vi "Get Row Subset as String Array.vi"(8 "error in (no error)":errorcluster, 9 "Replace FKs?":bool, 10 "Column Names (All)":string[](array[string]), 11 "Basic Table in":refnum<class "Basic Table.lvclass">) -> (0 "error out":errorcluster, 2 "Values":string[](array[string]), 3 "Basic Table out":refnum<class "Basic Table.lvclass">)   [LabVIEW 2020, in "Table.lvlib" / "Basic Table.lvclass"]
uses:
  Basic Table.lvclass
  Basic Table.lvclass/Basic Table.ctl
  Column Libraries/Column Interface/Column Interface Class/Column Interface.lvclass
  Table Configuration Interface/Table Configuration Interface.lvclass
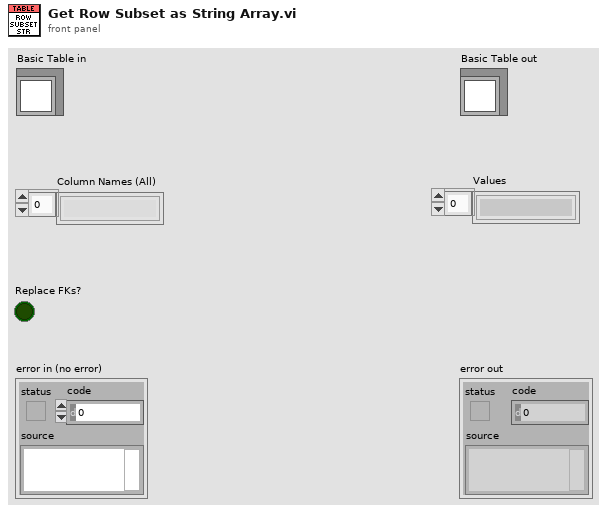
[diagram p1: front panel]
types:
  T1 = map{string, refnum<class "Column Interface.lvclass">}
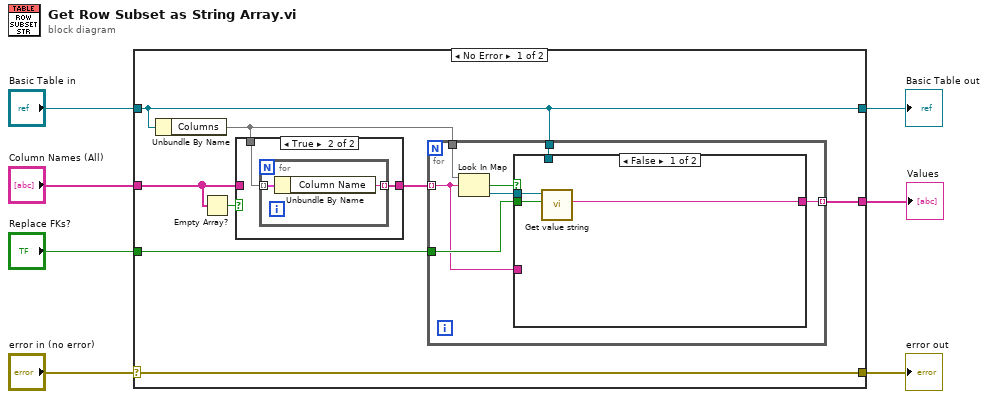
[diagram p0: block diagram]
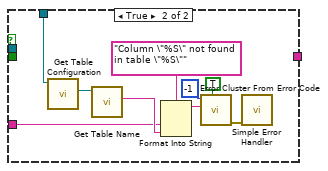
[diagram p3: hidden frame]
diagram:
  n1 = case shown="No Error" "error in (no error)" {
    selector: "error in (no error)" -> [w12 w41]
    tunnel: [w12 w41] -> w6
    tunnel: [w13 w40] -> w4
    tunnel: "Basic Table in" -> [w13 w40]
    tunnel: "Column Names (All)" -> [w10 _]
    tunnel: "Replace FKs?" -> [w15 _]
    tunnel: [w14 _] -> w1
    frame No Error {
      n2 = Unbundle By Name(w13) -> ("Columns"=w8:T1)
      n3 = Empty Array?(array=w10) -> (empty?=w11:bool)
      n4 = case shown="True" w11 {
        tunnel: w10 -> [w16 _]
        tunnel: [w16 w17] -> w9
        tunnel: w8 -> [_ w18]
        frame False {
        }
        frame True {
          n5 = for {
            tunnel: w18 -> [w20] mode=indexing
            tunnel: [w19] -> w17 mode=indexing
            n6 = Unbundle By Name(w20) -> ("Column Name"=w19:string)
          }
        }
      }
      n7 = for {
        tunnel: w9 -> [w22] mode=indexing
        tunnel: w15 -> [w25]
        tunnel: [w24] -> w14 mode=indexing
        tunnel: w13 -> [w23]
        tunnel: w8 -> [w21]
        n8 = Look In Map(map=w21, key=w22) -> (key not found?=w27:bool, value=w26:refnum<class "Column Interface.lvclass">)  [unwired: 1 in]
        n9 = case shown="False" w27 {
          tunnel: w26 -> [w30 _]
          tunnel: w25 -> [w29 _]
          tunnel: [w28 _] -> w24
          tunnel: w23 -> [_ w39]
          tunnel: w22 -> [_ w35]
          frame False {
            n10 = call-dynamic "Get value string.vi"("Replace FKs? (F)"=w29, "Column Interface in"=w30) -> ("Value"=w28:string)  [unwired: 6 in, 3 out]
          }
          frame True {
            n11 = call "Get Table Configuration.vi"("Basic Table in"=w39) -> ("Table Configuration"=w38:refnum<class "Table Configuration Interface.lvclass">)  [unwired: 8 in, 2 out]
            n12 = call-dynamic "Get Table Name.vi"("Table Configuration Interface in"=w38) -> ("Table Name"=w36:string)  [unwired: 8 in, 2 out]
            n13 = Format Into String(format string="Column \"%S\" not found in table \"%S\"", w35, w36) -> (resulting string=w34:string)  [unwired: 2 in, 1 out]
            n14 = call <vilib>:"Error Cluster From Error Code.vi"("show call chain? (False)"=TRUE, "error message (\"\")"=w34, "error code (0)"=-1) -> ("error out"=w33:errorcluster)  [unwired: 6 in]
            n15 = call <vilib>:"Simple Error Handler.vi"("error in (no error)"=w33) -> ()  [unwired: 4 in, 5 out]
          }
        }
      }
    }
    frame Error {
    }
  }
  "error out" <- w6
  "Basic Table out" <- w4
  "Values" <- w1
